vi "FTW-STR-ReplaceWhitespace.vi"(1 "Replace Spaces With...":string, 3 "Input":string) -> (0 "Output":string)   [LabVIEW 2013, in "XML.lvlib"]
uses:
  XML.lvlib
panel:
  # "Inputs"
  # "Outputs"
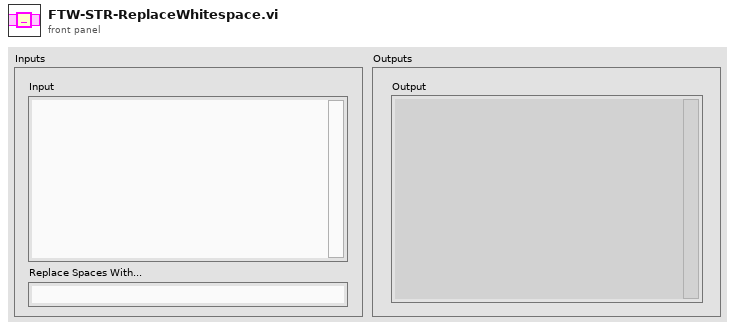
[diagram p1: front panel]
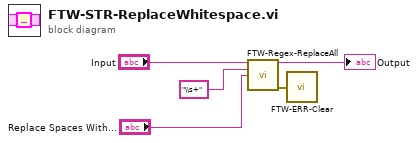
[diagram p0: block diagram]
diagram:
  n1 = call "FTW-Regex-ReplaceAll.vi"("String"="Input", "Search for (Regular Expression)"="\\s+" ("search string"), "Replace with"="Replace Spaces With...") -> ("String out"=→"Output":string, "error out"=w3:errorcluster)  [unwired: 10 in, 1 out]
  n2 = call "FTW-ERR-Clear.vi"("error to snuff"=w3) -> ()  [unwired: 1 out]
